vi "PCSLauncher.PC Launch PCS.vi"(0 "VI in":refnum<vi>, 5 "error in (no error)":errorcluster) -> (14 "VI out":refnum<vi>, 19 "error out":errorcluster)   [LabVIEW 2014, in "PCSLauncher.lvlib"]
uses:
  PCSLauncher.lvlib
  CS_Core/CSSystem/CSSystemLib/CSSystemLib.lvlib
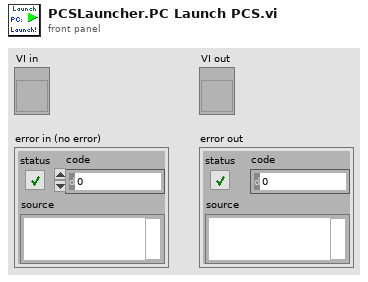
[diagram p1: front panel]
types:
  T1 = typedef "PCSLauncher.lvlib/PCSLauncher.i attribute.ctl" = cluster{"PCS Systems":cluster{"GUI Ref":refnum<vi>, "Super alive?":bool, "Start-GOG alive?":bool}[], "GUI Refs":cluster{"Delete":refnum<vi>, "Launch PCS":refnum<vi>}}
  T2 = cluster{"GUI Ref":refnum<vi>, "Super alive?":bool, "Start-GOG alive?":bool}[]
  T3 = enum8{"Enabled", "Disabled", "Disabled and Grayed Out"}
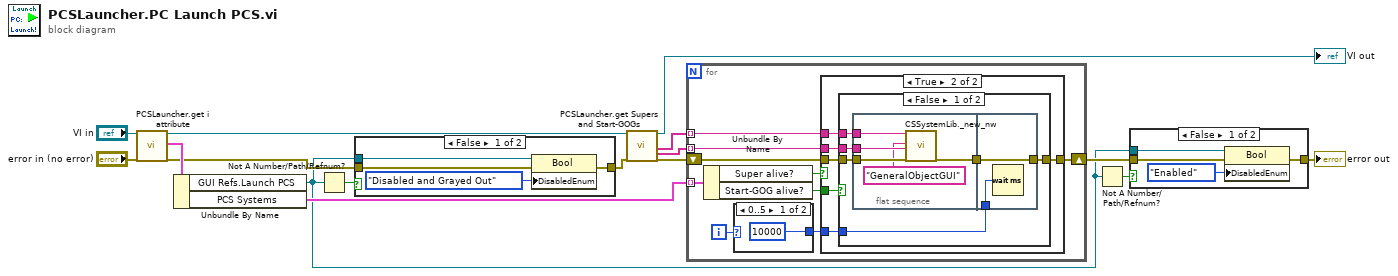
[diagram p0: block diagram]
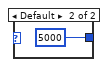
[diagram p4: hidden frame]
diagram:
  n1 = call "PCSLauncher.get i attribute.vi"("i ref in"="VI in", "error in (no error)"="error in (no error)") -> ("i ref out"=w11:refnum<vi>, "i attribute"=w16:T1, "error out"=w10:errorcluster)  [unwired: 15 in]
  n2 = Unbundle By Name(w16) -> ("GUI Refs.Launch PCS"=w1:refnum<vi>, "PCS Systems"=w15:T2)
  n3 = Not A Number/Path/Refnum?(number/path/refnum=w1) -> (NaN/Path/Refnum?=w5:bool)
  n4 = case shown="False" w5 {
    tunnel: w10 -> [w20 w21]
    tunnel: [w19 w21] -> w6
    tunnel: w1 -> [w18 _]
    frame False {
      n5 = property class="Bool"(reference=w18, error in=w20, "DisabledEnum"=T3."Disabled and Grayed Out" ("Disabled")) -> (error out=w19:errorcluster)  [unwired: 1 out]
    }
    frame True {
    }
  }
  n6 = call "PCSLauncher.get Supers and Start-GOGs.vi"("i ref in"=w11, "error in (no error)"=w6) -> ("i ref out"=→"VI out":refnum<vi>, "Start-GOG Instances"=w14:string[], "System Names"=w7:string[], "error out"=w9:errorcluster)  [unwired: 13 in, 1 out]
  n7 = for {
    tunnel: w15 -> [w30] mode=indexing
    shift-right: [w26] -> w4
    shift-left: w9 -> [w27]
    tunnel: w14 -> [w25] mode=indexing
    tunnel: w7 -> [w24] mode=indexing
    i -> [w23]
    n8 = Unbundle By Name(w30) -> ("Super alive?"=w29:bool, "Start-GOG alive?"=w28:bool)
    n9 = case shown="0..5" w23 {
      tunnel: [u32 10000 ("milliseconds to wait") u32 5000 ("milliseconds to wait")] -> w22
      frame 0..5 {
      }
      frame Default {
      }
    }
    n10 = case shown="True" w29 {
      tunnel: w28 -> [_ w37]
      tunnel: w27 -> [w33 w39]
      tunnel: [w33 w38] -> w26
      tunnel: w25 -> [_ w36]
      tunnel: w24 -> [_ w35]
      tunnel: w22 -> [_ w34]
      frame False {
      }
      frame True {
        n11 = case shown="False" w37 {
          tunnel: w39 -> [w45 w53]
          tunnel: [w44 w53] -> w38
          tunnel: w36 -> [w43 _]
          tunnel: w35 -> [w42 _]
          tunnel: w34 -> [w40 _]
          frame False {
            n12 = flat-sequence {
              tunnel: w45 -> [w50]
              tunnel: w43 -> [w48]
              tunnel: w42 -> [w47]
              tunnel: [w49] -> w41
              tunnel: [w52] -> w44
              tunnel: w41 -> [w52]
              tunnel: w40 -> [w51]
              frame #0 {
                n13 = call "CSSystemLib._new_nw.vi"("objectName"=w48, "className"="GeneralObjectGUI", "systemName"=w47, "error in (no error)"=w50) -> ("error out"=w49:errorcluster)  [unwired: 13 in, 2 out]
              }
              frame #1 {
                n14 = Wait (ms)(milliseconds to wait=w51) -> ()  [unwired: 1 out]
              }
            }
          }
          frame True {
          }
        }
      }
    }
  }
  n15 = Not A Number/Path/Refnum?(number/path/refnum=w1) -> (NaN/Path/Refnum?=w2:bool)
  n16 = case shown="False" w2 {
    tunnel: w4 -> [w57 w58]
    tunnel: [w56 w58] -> w3
    tunnel: w1 -> [w55 _]
    frame False {
      n17 = property class="Bool"(reference=w55, error in=w57, "DisabledEnum"=T3."Enabled" ("Disabled")) -> (error out=w56:errorcluster)  [unwired: 1 out]
    }
    frame True {
    }
  }
  "error out" <- w3
